vi "drawPosEstRobot.vi"(4 "Scale":dbl format="%#_13g", 6 "Offset":T1, 7 "Lado":enum16{"Esquerdo", "Direito"}(ring), 8 "error in (no error)":errorcluster, 9 "Robot":refnum<class "Robot.lvclass">, 10 "Picture In":picture, 11 "Vision in":refnum<class "Vision.lvclass">) -> (0 "error out":errorcluster, 2 "picture out":picture, 3 "Vision out":refnum<class "Vision.lvclass">)   [LabVIEW 2023, in "Vision.lvclass"]
uses:
  Vision.lvclass
  <vilib>/Utility/miscctls.llb/LVBoundsTypeDef.ctl
  Robot_class/Robot.lvclass
  C:/Users/lucio/Desktop/roboime/SSL_AI/Object_class/Object.lvclass
  Object_class/Object.lvclass/Object.ctl
  Robot_class/Robot.lvclass/Robot.ctl
  <vilib>/Analysis/coordinate.llb/2D Cartesian Coordinate Rotation (Scalar).vi
  Robot_class/Read orientation.vi
  Object_class/Read x.vi
  Object_class/Read y.vi
  Object_class/Read position(x,y).vi
  <vilib>/Analysis/NI_AALPro.lvlib
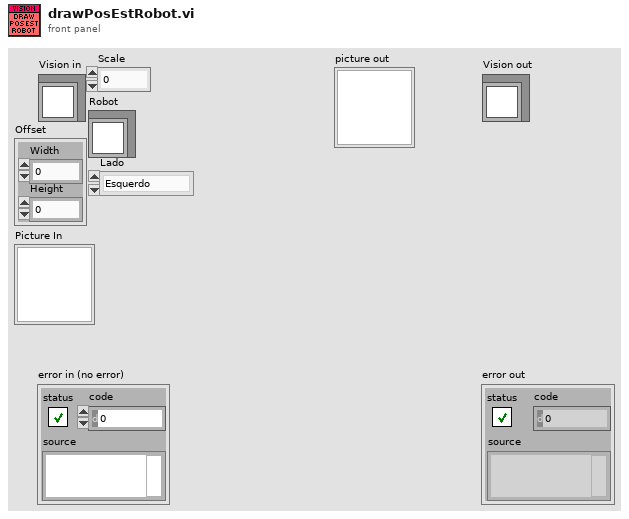
[diagram p1: front panel]
types:
  T1 = typedef "LVBoundsTypeDef.ctl" = cluster{"Width":u32, "Height":u32}
  T2 = cluster{"[0]":dbl, "[1]":dbl, "[2]":dbl, "[3]":dbl, "[4]":dbl, "[5]":dbl, "[6]":dbl, "[7]":dbl, "[8]":dbl}
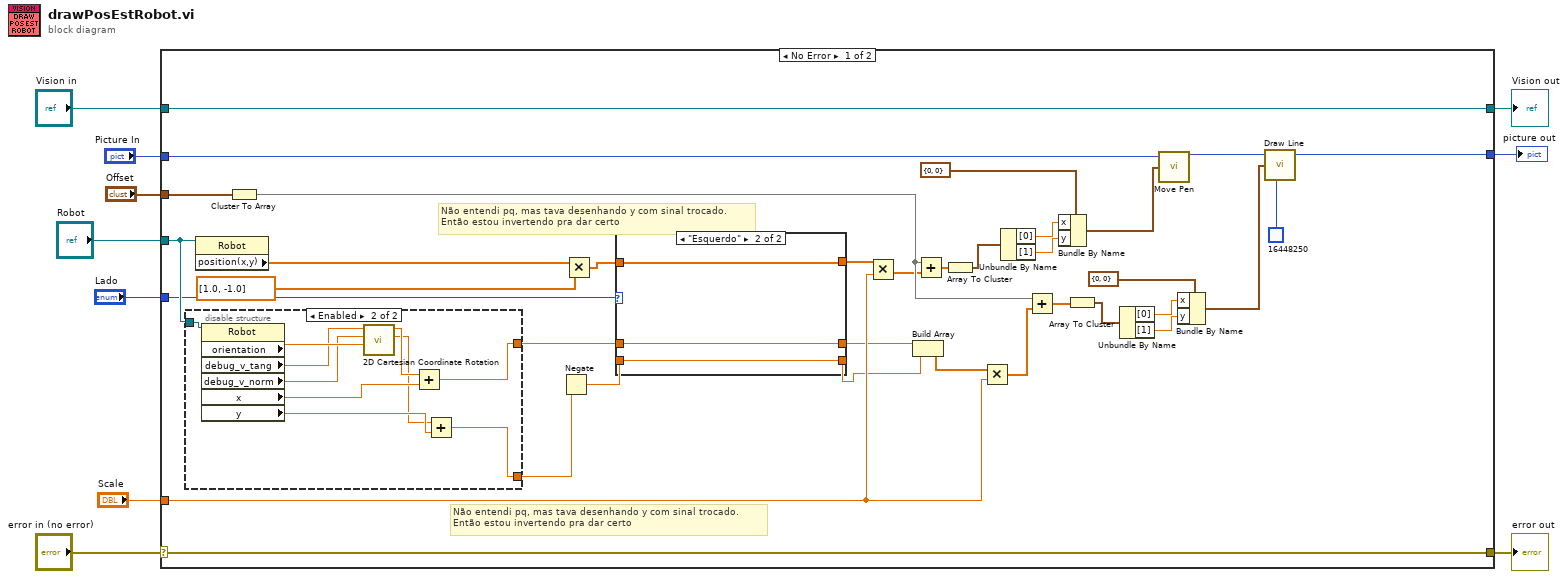
[diagram p0: block diagram]
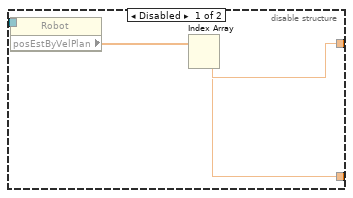
[diagram p2: hidden frame]
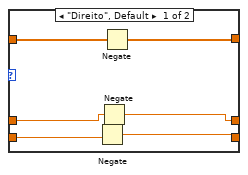
[diagram p3: hidden frame]
diagram:
  n1 = case shown="No Error" "error in (no error)" {
    selector: "error in (no error)" -> [w44 w70]
    tunnel: [w44 w70] -> w9
    tunnel: [w45 w69] -> w7
    tunnel: "Vision in" -> [w45 w69]
    tunnel: "Picture In" -> [w43 _]
    tunnel: "Robot" -> [w33 _]
    tunnel: "Offset" -> [w42 _]
    tunnel: [w34 _] -> w3
    tunnel: "Scale" -> [w23 _]
    tunnel: "Lado" -> [w17 _]
    frame No Error {
      # "Não entendi pq, mas tava desenhando y com sinal trocado.\nEntão estou invertendo pra dar certo"
      # "Não entendi pq, mas tava desenhando y com sinal trocado.\nEntão estou invertendo pra dar certo"
      n2 = disable-structure shown="Enabled" {
        disable-tunnel: w33 -> [w49 w59]
        disable-tunnel: [w47 w56] -> w12
        disable-tunnel: [w46 w55] -> w11
        frame Disabled {
          n3 = property class="Robot"(reference=w49) -> ("posEstByVelPlan"=w48:dbl[])  [unwired: 1 in, 2 out]
          n4 = Index Array(array=w48) -> (element #1=w47:dbl, element #2=w46:dbl)  [unwired: 2 in]
        }
        frame Enabled {
          n5 = property class="Robot"(reference=w59) -> ("orientation"=w54:dbl, "debug_v_tang"=w53:dbl, "debug_v_norm"=w52:dbl, "x"=w58:dbl, "y"=w57:dbl)  [unwired: 1 in, 2 out]
          n6 = call-poly <vilib>:"2D Cartesian Coordinate Rotation.vi"("theta"=w54, "y"=w52, "x"=w53) -> ("y out"=w50:dbl, "x out"=w51:dbl)  [unwired: 6 in, 1 out]
          n7 = Add(x=w51, y=w58) -> (x+y=w56:dbl)
          n8 = Add(x=w50, y=w57) -> (x+y=w55:dbl)
        }
      }
      n9 = property class="Robot"(reference=w33) -> ("position(x,y)"=w15:dbl[])  [unwired: 1 in, 2 out]
      n10 = Cluster To Array(cluster=w42) -> (array=w22:u32[])
      n11 = Negate(x=w11) -> (-x=w13:dbl)
      n12 = Multiply(x=w15, y=dbl[] [1.0, -1.0]) -> (x*y=w16:dbl[])
      n13 = case shown="\"Esquerdo\"" w17 {
        tunnel: [w65 w66] -> w20
        tunnel: [w61 w68] -> w19
        tunnel: w12 -> [w62 w68]
        tunnel: w13 -> [w64 w67]
        tunnel: [w63 w67] -> w18
        tunnel: w16 -> [w60 w66]
        frame "Direito", Default {
          n14 = Negate(x=w64) -> (-x=w63:dbl)
          n15 = Negate(x=w62) -> (-x=w61:dbl)
          n16 = Negate(x=w60) -> (-x=w65:dbl[])
        }
        frame "Esquerdo" {
        }
      }
      n17 = Multiply(x=w20, y=w23) -> (x*y=w21:dbl[])
      n18 = Build Array(w19, w18) -> (w32:dbl[])
      n19 = Add(x=w22, y=w21) -> (x+y=w41:dbl[])
      n20 = Array To Cluster(array=w41) -> (cluster=w39:T2)
      n21 = Multiply(x=w32, y=w23) -> (x*y=w31:dbl[])
      n22 = Unbundle By Name(w39) -> ("[0]"=w38:dbl, "[1]"=w37:dbl)
      n23 = Add(x=w22, y=w31) -> (x+y=w27:dbl[])
      n24 = Bundle By Name(cluster=cluster{"x":i16, "y":i16} {"x"=0, "y"=0} ("new position"), "x"=w38, "y"=w37) -> (w36:cluster{"x":i16, "y":i16})
      n25 = Array To Cluster(array=w27) -> (cluster=w26:T2)
      n26 = Unbundle By Name(w26) -> ("[0]"=w30:dbl, "[1]"=w29:dbl)
      n27 = call <vilib>:"Move Pen.vi"("new position"=w36, "picture"=w43) -> ("new picture"=w35:picture)  [unwired: 3 in]
      n28 = Bundle By Name(cluster=cluster{"x":i16, "y":i16} {"x"=0, "y"=0} ("new position"), "x"=w30, "y"=w29) -> (w25:cluster{"x":i16, "y":i16})
      n29 = call <vilib>:"Draw Line.vi"("picture"=w35, "end point"=w25, "color(black)"=u32 16448250) -> ("new picture"=w34:picture)  [unwired: 6 in]
    }
    frame Error {
    }
  }
  "error out" <- w9
  "Vision out" <- w7
  "picture out" <- w3
